vi "uPolicy_TopicIsRelevant.vi"(8 "error in (no error)":errorcluster, 10 "Observed Topic (Lower Case)":string, 11 "SingleTopic in":refnum<class "SingleTopic.lvclass">) -> (0 "error out":errorcluster, 2 "Relevant?":bool, 3 "SingleTopic out":refnum<class "SingleTopic.lvclass">)   [LabVIEW 2023, in "uFramework_pack_uPolicy.lvlib" / "SingleTopic.lvclass"]
uses:
  SingleTopic.lvclass
  SingleTopic.lvclass/SingleTopic.ctl
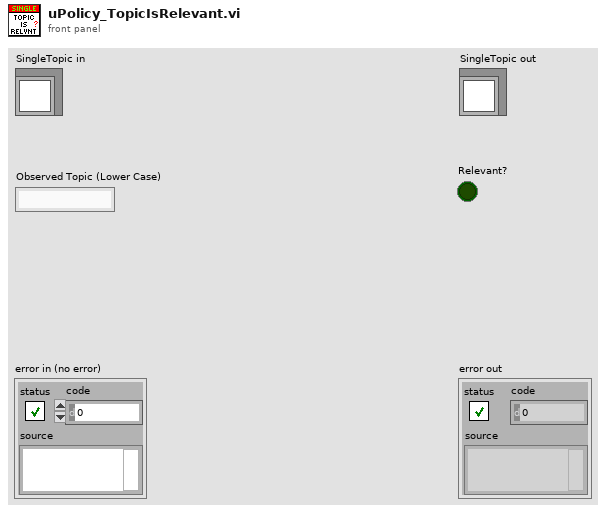
[diagram p1: front panel]
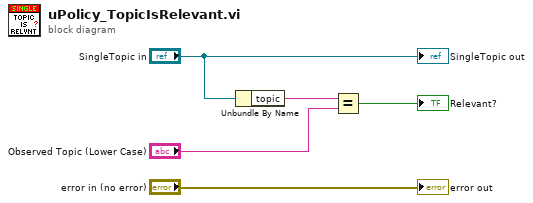
[diagram p0: block diagram]
diagram:
  n1 = Unbundle By Name("SingleTopic in") -> ("topic"=w3:string)
  n2 = Equal?(x=w3, y="Observed Topic (Lower Case)") -> (x = y?=→"Relevant?":bool)
  "error out" <- "error in (no error)"
  "SingleTopic out" <- "SingleTopic in"
